vi "GetDateTimeString.vi"(8 "error in (no error)":errorcluster, 11 "Generator in":refnum<class "Generator.lvclass">) -> (0 "error out":errorcluster, 3 "Generator out":refnum<class "Generator.lvclass">)   [LabVIEW 2014, in "Generator.lvlib" / "Generator.lvclass"]
uses:
  Generator.lvclass
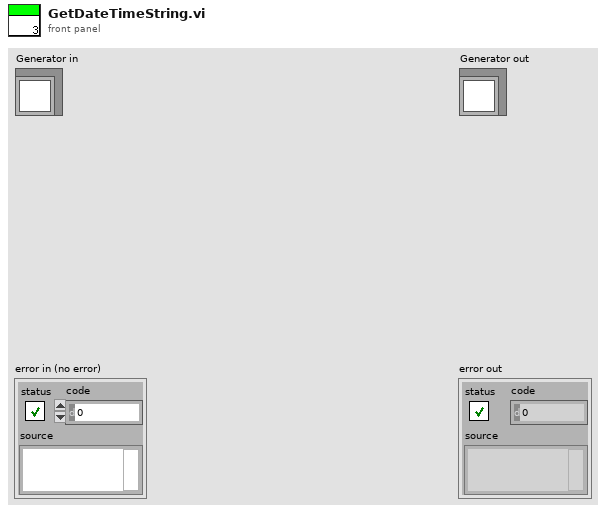
[diagram p1: front panel]
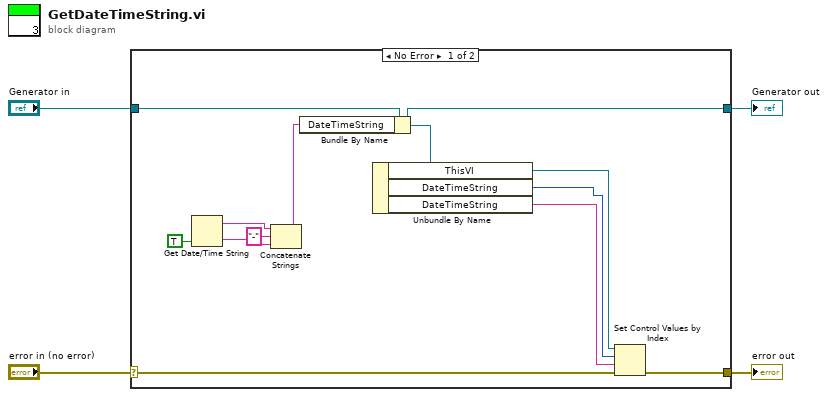
[diagram p0: block diagram]
diagram:
  n1 = case shown="No Error" "error in (no error)" {
    selector: "error in (no error)" -> [w15 w18]
    tunnel: [w9 w18] -> w3
    tunnel: [w8 w17] -> w1
    tunnel: "Generator in" -> [w16 w17]
    frame No Error {
      n2 = Get Date/Time String(want seconds? (F)=TRUE) -> (date string=w13:string, time string=w12:string)  [unwired: 2 in]
      n3 = Concatenate Strings(w13, "-" ("string"), w12) -> (w10:string)
      n4 = Bundle By Name(cluster=w16, "DateTimeString"=w10) -> (w8:refnum<class "Generator.lvclass">)
      n5 = Unbundle By Name(w8) -> ("ThisVI"=w7:refnum<vi>, "DateTimeString"=w6:i32, "DateTimeString"=w5:string)
      n6 = Set Control Values by Index(0:w7, 1:w6, 2:w5, 3:w15) -> (11:w9:errorcluster)
    }
    frame Error {
    }
  }
  "error out" <- w3
  "Generator out" <- w1
